vi "Sel_match_from_StringArr.vi"(7 "Ignore case (TRUE def)":bool=TRUE, 10 "String to match":string="c:\\DATA", 11 "String Array In":string[](array[string])=["the settings file open properly", "Init", "the temperature file open properly", "astrocamInit: lodFile = C:\\vlt\\assembly\\h2rg-20141010\\SNAP\\tim_h2rg_SNAP.lod", "Getting device bindings ... done !", "Opening PCI driver ... ", "done!", "Calling astrocamConfig ", "astrocamConfig start ...", "Setting up controllerdone!", "Opening shutter ...", "Configuring ...", "RNT = 1", "OFA 0x1ec", "Waiting for image ..", "Done=true ", "GotImage - returning  ", "c:\\DATA\\20141011-102717-0.fits", "Got image.", "Waiting for image ..", "Done=true ", "GotImage - returning  ", "c:\\DATA\\20141011-102717-1.fits", "Got image.", "Close", "Test", "Done", ""]) -> (1 "Inx Exact match":i32[](array[numeric]), 2 "Inx matches":i32[](array[numeric]), 3 "String Array Matched":string[](array[string])=["c:\\DATA\\20141011-102717-0.fits", "c:\\DATA\\20141011-102717-1.fits"], 4 "String Found Arr":bool[](array[boolean]), 5 "Str found?":bool)   [LabVIEW 2019]
panel:
  out "Array Size":i32=2
  out "String Found Inx":i32[](array[numeric])=[-1, -1, -1, -1, -1, -1, -1, -1, -1, -1, -1, -1, -1, -1, -1, -1, -1, 0, -1, -1, -1, -1, 0, -1, -1, -1, -1, -1]
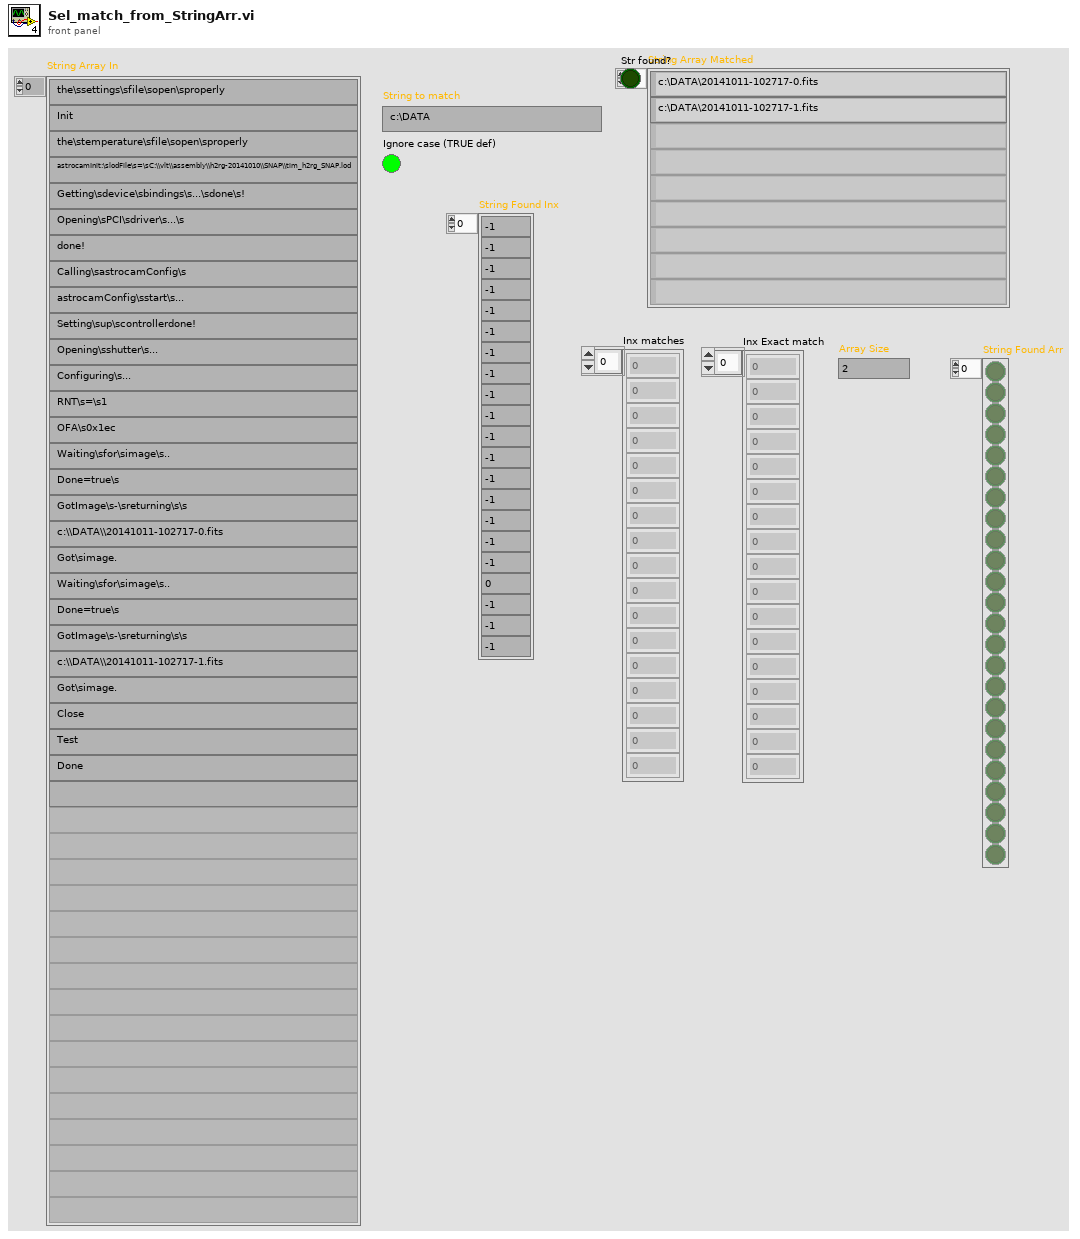
[diagram p1: front panel]
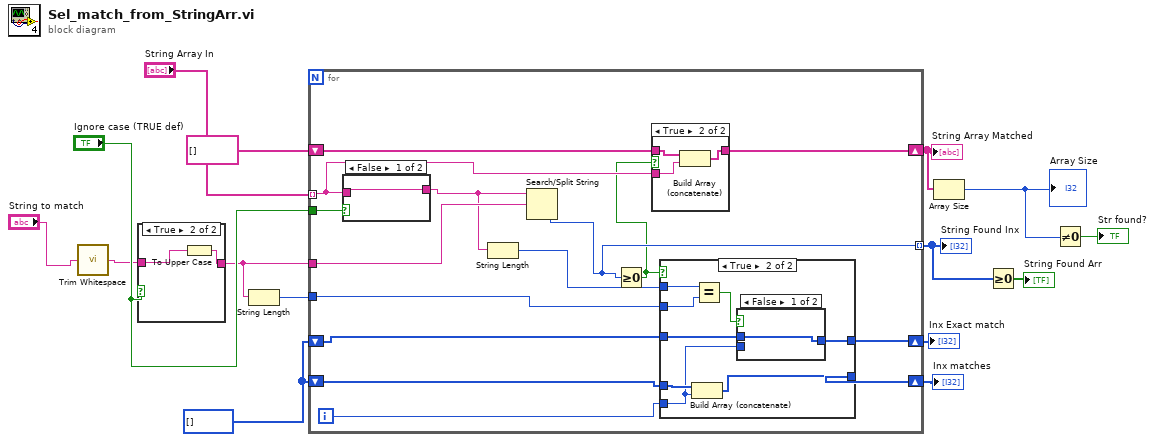
[diagram p0: block diagram]
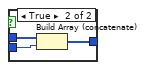
[diagram p4: hidden frame]
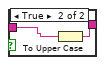
[diagram p5: hidden frame]
diagram:
  w6 = i32[] []
  n1 = call <vilib>:"Trim Whitespace.vi"("string"="String to match") -> ("trimmed string"=w10:string)  [unwired: 1 in]
  n2 = case shown="True" "Ignore case (TRUE def)" {
    tunnel: w10 -> [w16 w18]
    tunnel: [w16 w17] -> w9
    frame False {
    }
    frame True {
      n3 = To Upper Case(1:w18) -> (0:w17:string)
    }
  }
  n4 = String Length(string=w9) -> (length=w8:i32)
  n5 = for {
    tunnel: "String Array In" -> [w30] mode=indexing
    shift-right: [w33] -> w14
    shift-left: string[] [] -> [w32]
    tunnel: [w31] -> w2 mode=indexing
    tunnel: "Ignore case (TRUE def)" -> [w29]
    tunnel: w9 -> [w28]
    shift-right: [w21] -> w7
    shift-left: w6 -> [w25]
    tunnel: w8 -> [w24]
    shift-right: [w19] -> w5
    shift-left: w6 -> [w20]
    i -> [w26]
    n6 = case shown="False" w29 {
      tunnel: w30 -> [w48 w50]
      tunnel: [w48 w49] -> w23
      frame False {
      }
      frame True {
        n7 = To Upper Case(1:w50) -> (0:w49:string)
      }
    }
    n8 = String Length(string=w23) -> (length=w22:i32)
    n9 = Search/Split String(string=w23, search string/char (-)=w28) -> (offset of match=w31:i32)  [unwired: 1 in, 2 out]
    n10 = Greater Or Equal To 0?(x=w31) -> (x >= 0?=w27:bool)
    n11 = case shown="True" w27 {
      tunnel: w30 -> [_ w54]
      tunnel: [w51 w53] -> w33
      tunnel: w32 -> [w51 w52]
      frame False {
      }
      frame True {
        n12 = Build Array (concatenate)(w52, w54) -> (w53:string[])
      }
    }
    n13 = case shown="True" w27 {
      tunnel: [w35 w43] -> w21
      tunnel: w25 -> [w35 w42]
      tunnel: w26 -> [_ w36]
      tunnel: w24 -> [_ w40]
      tunnel: w22 -> [_ w41]
      tunnel: w20 -> [w34 w38]
      tunnel: [w34 w37] -> w19
      frame False {
      }
      frame True {
        n14 = Build Array (concatenate)(w42, w36) -> (w43:i32[])
        n15 = Equal?(x=w41, y=w40) -> (x = y?=w39:bool)
        n16 = case shown="False" w39 {
          tunnel: w38 -> [w44 w47]
          tunnel: [w44 w46] -> w37
          tunnel: w36 -> [_ w45]
          frame False {
          }
          frame True {
            n17 = Build Array (concatenate)(w47, w45) -> (w46:i32[])
          }
        }
      }
    }
  }
  "String Array Matched" <- w14
  "String Found Inx" <- w2
  "Inx matches" <- w7
  "Inx Exact match" <- w5
  n18 = Array Size(array=w14) -> (size(s)=w4:i32)
  "Array Size" <- w4
  n19 = Greater Or Equal To 0?(x=w2) -> (x >= 0?=→"String Found Arr":bool[])
  n20 = Not Equal To 0?(x=w4) -> (x != 0?=→"Str found?":bool)
